vi "test_VariousDataTypes_GetParametersAndCheckDataTypes_InvalidParameterNamesMatch.vi"(8 "error in":errorcluster) -> (0 "error out":errorcluster, 2 "result":string, 3 "pass":bool)   [LabVIEW 2020, in "MeasurementServerTests.lvlib"]
uses:
  MeasurementServerTests.lvlib
  Runtime/Measurements/Plug-In SDK Measurement.lvlib
  gRPC/Generated APIs/ni/protobuf/types/RPC Messages/ni_protobuf_types_DoubleXYData.ctl
  gRPC/Generated APIs/ni/protobuf/types/ni.protobuf.types.lvlib
panel:
  out "actual invalid names":string[](array[string])
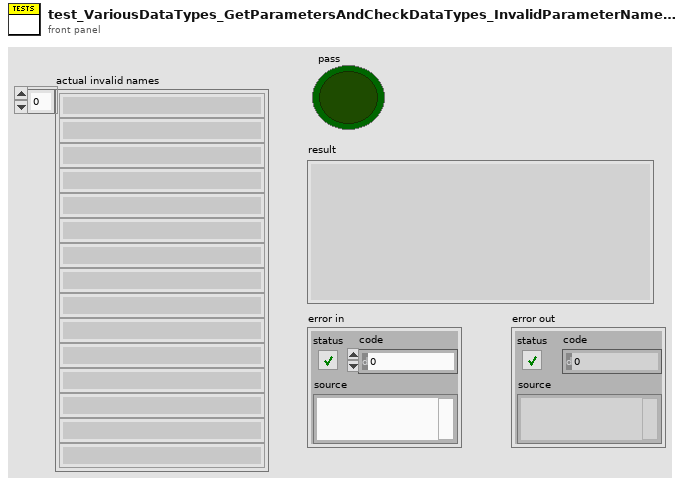
[diagram p1: front panel]
types:
  T1 = typedef "ni.protobuf.types.lvlib/ni_protobuf_types_DoubleXYData.ctl" = cluster{"x_data":dbl[], "y_data":dbl[]}
  T2 = cluster{"double":dbl, "int64":i64, "uint64":u64, "int32":i32, "uint32":u32, "int16":i16, "uint16":u16, "bool":bool, "string":string, "double array":dbl[], "uint64 array":u64[], "ni_protobuf_types_DoubleXYData":T1, "cluster of double":cluster{"Numeric":dbl}, "enum u32":enum32{""}, "enum u16":enum16{""}, "enum u8":enum8{""}}
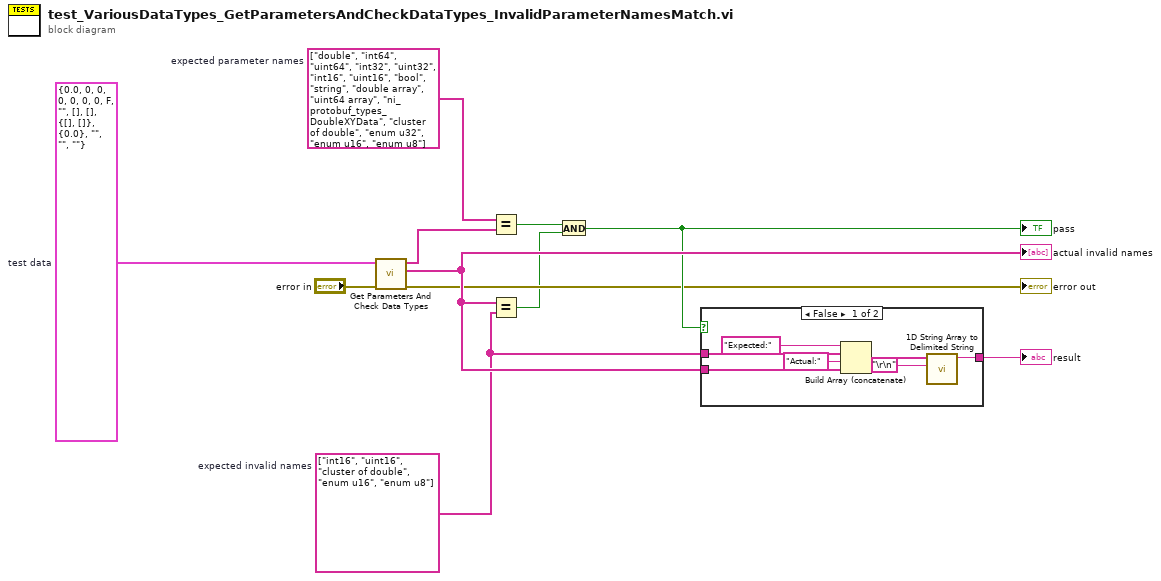
[diagram p0: block diagram]
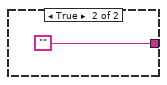
[diagram p2: hidden frame]
diagram:
  w1 = string[] ["double", "int64", "uint64", "int32", "uint32", "int16", "uint16", "bool", "string", "double array", "uint64 array", "ni_protobuf_types_DoubleXYData", "cluster of double", "enum u32", "enum u16", "enum u8"]  # expected parameter names
  w4 = T2 {"double"=0.0, "int64"=0, "uint64"=0, "int32"=0, "uint32"=0, "int16"=0, "uint16"=0, "bool"=FALSE, "string"="", "double array"=[], "uint64 array"=[], "ni_protobuf_types_DoubleXYData"={"x_data"=[], "y_data"=[]}, "cluster of double"={"Numeric"=0.0}, "enum u32"=enum."", "enum u16"=enum."", "enum u8"=enum.""}  # test data
  w2 = string[] ["int16", "uint16", "cluster of double", "enum u16", "enum u8"]  # expected invalid names
  n1 = call "Get Parameters And Check Data Types.vi"("error in"="error in", "variant"=w4) -> ("error out"=→"error out":errorcluster, "parameters with invalid type"=w11:string[], "parameter names"=w3:string[])  [unwired: 7 in]
  "actual invalid names" <- w11
  n2 = Equal?(x=w1, y=w3) -> (x = y?=w6:bool)
  n3 = Equal?(x=w11, y=w2) -> (x = y?=w5:bool)
  n4 = And(x=w6, y=w5) -> (x .and. y?=w9:bool)
  "pass" <- w9
  n5 = case shown="False" w9 {
    tunnel: w11 -> [w18 _]
    tunnel: [w13 ""] -> w8
    tunnel: w2 -> [w12 _]
    frame False {
      n6 = Build Array (concatenate)("Expected:", w12, "Actual:", w18) -> (w15:string[])
      n7 = call <vilib>:"1D String Array to Delimited String.vi"("delimiter"="\r\n", "string array"=w15) -> ("delimited string"=w13:string)  [unwired: 9 in]
    }
    frame True {
    }
  }
  "result" <- w8
